vi "4-1.vi"() -> ()   [LabVIEW 2022 SP3, in "AoC22.lvlib"]
uses:
  AoC22.lvlib
  <vilib>/IlluminatedG/lv-stream/Stream.lvlib
panel:
  out "Numeric":i32
  out "Array":i32[][](array[numeric])
  out "sum":i16
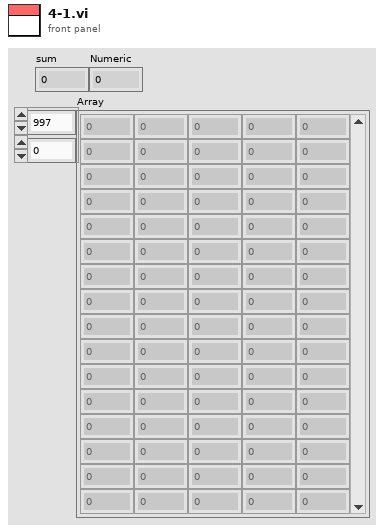
[diagram p1: front panel]
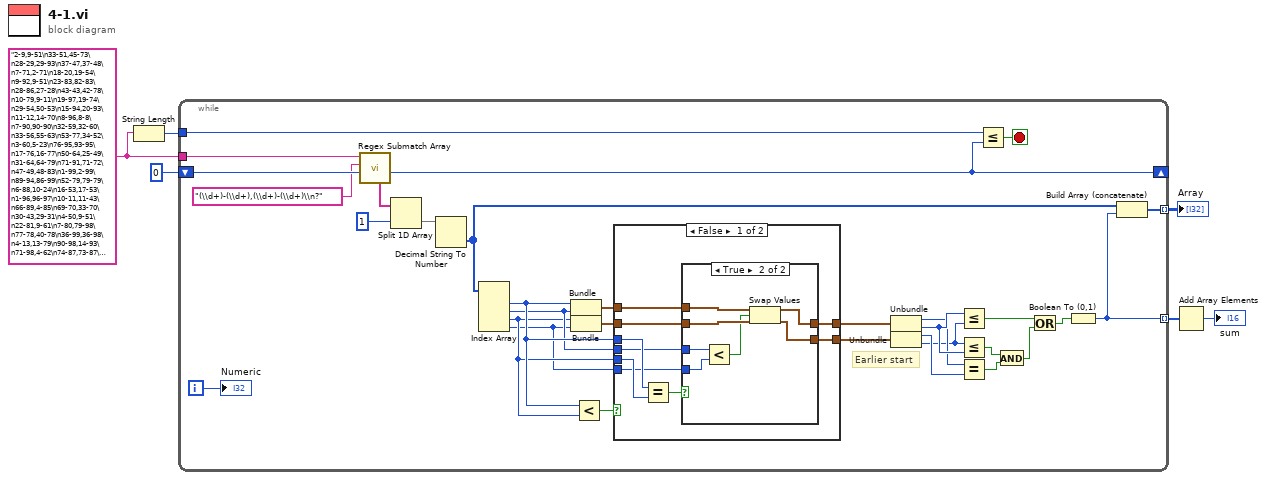
[diagram p0: block diagram]
diagram:
  w5 = "2-9,9-51\n33-51,45-73\n28-29,29-93\n37-47,37-48\n7-71,2-71\n18-20,19-54\n9-92,9-51\n23-83,82-83\n28-86,27-28\n43-43,42-78\n10-79,9-11\n19-97,19-74\n29-54,50-53\n15-94,20-93\n11-12,14-70\n8-96,8-8\n7-90,90-90\n32-59,32-60\n33-56,55-63\n53-77,34-52\n3-60,5-23\n76-95,93-95\n17-76,16-77\n50-64,25-49\n31-64,64-79\n71-91,71-72\n47-49,48-83\n1-99,2-99\n89-94,86-99\n52-79,79-79\n6-88,10-24\n16-53,17-53\n1-96,96-97\n10-11,11-43\n66-89,4-85\n69-70,33-70\n30-43,29-31\n4-50,9-51\n22-81,9-61\n7-80,79-98\n77-78,40-78\n36-99,36-98\n4-13,13-79\n90-98,14-93\n71-98,4-62\n74-87,73-87\n46-86,84-97\n1-57,36-58\n82-96,9-83\n27-96,2-96\n33-33,33-33\n93-94,45-94\n92-92,4-93\n3-70,1-77\n53-94,72-86\n84-85,39-85\n10-74,10-88\n59-95,72-83\n37-75,23-85\n17-19,10-19\n1-83,1-82\n2-93,94-94\n26-84,83-84\n35-57,34-58\n16-74,17-17\n38-88,38-89\n70-96,69-96\n43-76,77-88\n2-99,2-87\n33-56,74-81\n19-50,19-20\n26-94,94-97\n5-78,2-82\n27-77,26-77\n47-98,45-99\n6-89,5-5\n35-56,22-57\n3-96,1-3\n97-97,24-96\n4-35,5-68\n3-5,34-85\n89-90,82-91\n6-46,6-65\n17-34,17-35\n10-82,11-81\n4-53,2-4\n21-88,21-75\n67-99,22-68\n3-89,90-94\n4-97,2-98\n2-69,2-3\n41-62,42-61\n39-88,10-90\n3-43,18-42\n3-83,28-84\n74-87,22-86\n35-98,35-99\n11-92,10-10\n8-15,9-17\n10-17,55-94\n54-74,53-60\n3-96,3-4\n5-18,5-70\n6-88,3-3\n98-98,5-99\n60-87,59-84\n28-76,27-77\n17-26,26-70\n4-6,3-5\n83-99,83-97\n10-65,65-69\n6-73,2-74\n44-96,44-95\n89-89,10-88\n2-91,95-96\n13-60,12-59\n6-29,5-27\n57-57,12-58\n48-85,48-85\n97-98,20-85\n62-97,99-99\n3-6,8-99\n20-34,12-14\n18-84,17-85\n5-88,4-46\n63-67,32-64\n52-80,52-80\n35-97,3-9\n35-78,35-79\n42-65,66-66\n30-30,30-93\n35-44,36-41\n26-95,4-92\n5-5,5-30\n15-88,16-87\n14-54,55-55\n8-41,41-57\n11-93,20-84\n7-61,6-7\n16-37,37-89\n36-89,35-90\n9-39,9-40\n79-92,72-80\n39-97,97-98\n75-81,21-76\n3-70,71-71\n2-94,2-94\n4-5,5-80\n2-84,2-84\n44-57,45-56\n36-76,3-77\n48-54,53-98\n14-71,3-71\n18-98,2-98\n29-85,14-30\n5-88,4-6\n54-84,22-53\n11-75,61-79\n73-74,39-73\n61-98,61-62\n1-4,5-59\n66-94,88-94\n32-38,38-64\n4-59,1-5\n25-57,24-36\n45-69,46-68\n53-77,53-63\n1-94,4-93\n17-89,88-90\n9-90,21-39\n9-90,8-15\n65-82,66-81\n7-83,7-83\n24-98,24-77\n1-1,3-99\n16-18,17-47\n31-87,32-88\n96-98,34-95\n32-67,31-67\n16-58,57-57\n37-83,24-40\n4-66,3-66\n36-74,44-73\n22-81,22-23\n2-7,7-61\n20-21,21-76\n74-74,7-73\n12-46,4-11\n95-99,16-96\n38-80,39-39\n1-19,7-65\n39-53,39-84\n24-82,23-28\n43-44,43-92\n48-60,49-94\n66-85,31-65\n30-31,30-64\n56-95,36-55\n68-93,58-68\n47-59,46-46\n12-33,32-97\n57-75,62-84\n7-8,12-93\n42-75,76-76\n33-81,34-80\n4-5,4-97\n56-78,23-95\n53-53,54-67\n6-46,10-77\n55-87,87-88\n63-83,63-63\n1-1,1-43\n80-92,49-92\n95-99,11-95\n31-34,36-46\n25-83,84-96\n2-98,3-98\n1-3,2-69\n83-97,52-97\n35-93,37-78\n15-44,45-45\n1-99,2-99\n65-89,8-95\n23-59,28-60\n94-94,18-93\n3-44,12-90\n14-51,5-51\n13-38,12-14\n50-88,49-89\n46-69,47-47\n38-44,44-53\n11-73,87-88\n3-58,2-3\n42-89,90-98\n5-41,6-36\n48-90,47-49\n14-50,14-50\n16-24,3-16\n40-41,40-48\n37-37,1-38\n6-38,26-38\n8-96,17-95\n13-98,99-99\n2-57,3-56\n3-30,1-37\n4-68,4-67\n17-20,21-90\n13-17,16-23\n24-25,25-92\n2-2,1-96\n19-91,90-93\n6-79,7-50\n27-28,22-28\n12-98,9-98\n1-4,3-71\n10-20,19-51\n15-15,15-66\n95-95,30-96\n1-93,3-90\n41-43,42-86\n77-93,76-77\n87-99,96-99\n1-99,98-98\n13-70,2-64\n66-84,51-67\n24-89,43-92\n3-43,2-4\n46-48,47-82\n6-96,1-5\n13-76,13-76\n1-83,84-96\n42-60,3-21\n10-49,5-16\n42-95,96-97\n35-35,32-34\n5-7,6-27\n6-16,30-46\n98-99,14-97\n23-75,22-24\n16-18,17-90\n72-73,57-71\n13-78,10-98\n57-62,58-66\n22-57,58-58\n2-75,5-72\n7-24,11-66\n37-91,68-90\n57-94,6-93\n57-67,57-68\n6-18,17-85\n10-10,11-73\n19-35,34-34\n13-30,29-71\n78-78,68-79\n40-54,40-40\n14-60,13-60\n6-31,31-94\n25-76,55-75\n76-81,47-81\n34-58,43-57\n16-60,15-17\n95-97,9-96\n6-7,7-87\n99-99,3-98\n13-36,28-69\n13-26,12-26\n17-57,56-58\n20-95,27-44\n81-88,81-88\n29-45,28-45\n71-77,71-78\n4-17,28-82\n75-77,12-76\n40-44,39-41\n60-90,89-89\n28-43,28-48\n8-89,74-90\n1-4,6-77\n7-74,75-75\n84-94,6-93\n94-95,21-95\n10-63,64-87\n23-97,25-83\n11-68,11-74\n41-45,40-44\n30-88,83-87\n26-74,67-68\n2-6,7-60\n41-41,31-37\n91-91,20-90\n8-8,7-77\n66-77,74-77\n89-97,92-99\n63-70,64-70\n95-98,3-96\n14-79,78-78\n58-81,80-92\n59-94,58-58\n12-23,13-83\n9-85,9-9\n13-97,9-92\n56-73,16-57\n2-96,99-99\n31-73,30-41\n17-91,18-90\n74-94,64-75\n8-97,1-4\n6-95,5-6\n94-97,38-95\n9-80,53-69\n8-8,8-70\n11-94,11-93\n38-86,87-93\n7-85,6-7\n3-90,1-98\n18-88,14-73\n7-95,8-94\n27-77,7-26\n55-98,55-56\n49-90,85-91\n14-64,14-37\n91-95,8-92\n48-94,10-48\n95-96,68-95\n84-98,82-84\n69-69,13-68\n23-93,11-24\n8-25,25-30\n15-79,14-16\n2-98,1-97\n60-70,59-70\n11-69,68-74\n56-83,32-82\n18-97,18-97\n30-72,57-71\n10-55,14-69\n9-9,9-96\n20-92,6-19\n17-47,19-73\n51-86,85-85\n94-94,3-95\n1-99,99-99\n19-22,18-22\n51-76,50-52\n99-99,19-98\n95-95,24-46\n35-81,36-66\n25-86,29-87\n6-50,4-94\n12-35,56-70\n15-69,70-70\n6-95,96-97\n84-97,75-96\n10-10,10-10\n2-22,13-23\n43-90,91-91\n2-95,1-3\n25-65,25-25\n3-57,3-21\n50-64,38-50\n9-94,93-96\n6-49,7-48\n69-82,73-83\n74-95,71-95\n8-95,9-94\n36-78,37-77\n29-31,30-86\n7-78,26-77\n66-66,38-67\n43-86,44-92\n29-31,30-84\n15-59,58-84\n1-1,3-98\n14-33,20-34\n80-80,45-79\n35-95,23-73\n14-16,15-56\n3-56,1-57\n5-98,98-98\n80-93,13-90\n49-96,95-98\n2-85,1-84\n36-43,35-79\n4-99,2-99\n29-94,29-94\n1-95,96-96\n42-47,43-91\n35-98,31-39\n48-71,14-36\n10-70,71-99\n3-3,3-52\n89-89,58-88\n2-91,1-92\n60-82,40-61\n49-50,49-91\n97-97,1-94\n9-9,9-45\n1-1,3-40\n1-99,8-98\n61-63,60-63\n11-38,38-59\n8-54,3-5\n72-80,72-79\n30-97,30-96\n1-99,2-99\n14-62,49-61\n15-28,14-54\n20-27,27-87\n5-55,5-97\n1-94,69-94\n95-98,16-96\n62-62,61-76\n2-10,4-53\n8-73,7-73\n4-87,94-97\n10-82,10-84\n11-77,77-78\n6-98,6-6\n44-63,44-52\n58-90,57-58\n15-79,16-79\n3-8,4-72\n7-17,8-49\n19-87,18-20\n94-94,14-95\n47-65,66-66\n82-97,82-82\n2-11,6-12\n34-36,18-73\n1-30,27-31\n5-97,4-91\n33-83,9-33\n21-73,72-74\n9-75,8-89\n3-6,5-93\n3-77,1-4\n4-31,8-92\n42-50,41-51\n72-89,60-85\n86-89,14-85\n13-72,12-72\n67-79,37-79\n97-99,9-97\n9-50,8-88\n44-65,44-44\n47-78,79-91\n24-64,12-32\n8-83,9-82\n18-85,5-86\n4-69,5-70\n5-91,7-98\n17-19,4-19\n80-80,1-81\n1-95,4-94\n1-69,4-34\n58-59,58-62\n83-95,30-84\n2-30,3-91\n11-30,29-61\n5-94,8-93\n8-12,12-96\n78-95,36-79\n15-87,83-88\n84-84,84-84\n8-10,9-81\n79-98,26-98\n2-2,2-94\n62-78,46-62\n2-79,1-3\n73-75,3-73\n52-54,35-53\n46-81,4-82\n9-96,9-9\n68-98,97-99\n29-74,6-30\n31-31,32-67\n2-97,1-3\n43-47,17-44\n31-75,69-86\n60-72,23-71\n10-67,10-68\n61-63,4-62\n26-65,50-65\n9-29,35-88\n14-78,15-78\n4-76,77-90\n32-33,64-78\n52-92,53-97\n29-47,24-45\n52-70,53-69\n96-96,15-97\n52-89,46-89\n3-5,6-84\n12-75,12-81\n46-57,28-46\n53-76,14-57\n18-52,52-89\n33-53,71-92\n12-28,29-67\n3-7,4-52\n50-55,55-66\n63-63,63-92\n12-86,12-86\n44-57,43-44\n2-61,3-61\n56-85,1-57\n4-6,6-98\n1-75,56-75\n58-60,59-59\n4-22,15-23\n4-17,2-4\n1-33,2-32\n10-89,20-90\n8-72,2-73\n10-69,10-45\n65-80,50-80\n22-94,22-75\n24-98,24-99\n23-99,26-98\n6-71,1-83\n4-5,4-97\n5-25,14-43\n23-74,22-87\n89-96,97-99\n41-46,26-45\n20-86,20-95\n9-97,9-96\n74-77,30-82\n56-68,58-69\n7-10,7-94\n2-87,87-93\n49-92,72-91\n13-14,13-72\n37-38,37-39\n56-74,7-73\n17-95,51-99\n10-95,10-10\n1-97,96-98\n23-53,27-69\n29-65,29-58\n32-89,31-32\n25-43,25-26\n60-61,61-91\n87-89,33-88\n35-35,35-37\n11-47,39-62\n50-52,28-51\n65-65,20-64\n34-91,40-59\n10-67,99-99\n5-82,4-6\n11-40,11-11\n17-57,1-18\n21-22,21-93\n6-79,6-7\n1-75,75-92\n3-82,4-70\n29-58,29-82\n33-33,33-62\n25-33,24-25\n8-80,9-9\n45-69,44-64\n13-17,17-37\n2-97,2-98\n13-88,12-14\n3-61,16-69\n4-95,1-2\n43-45,44-81\n24-71,70-70\n55-92,91-97\n93-98,20-92\n51-52,36-52\n1-97,20-98\n1-86,1-86\n41-85,86-97\n26-28,26-29\n11-38,10-39\n32-70,31-31\n29-31,30-86\n68-94,84-94\n14-19,19-71\n39-94,94-97\n20-41,40-51\n3-88,89-98\n65-86,79-85\n38-99,38-39\n64-75,64-65\n90-92,6-91\n4-30,6-29\n3-47,2-48\n72-85,71-81\n64-70,65-65\n26-95,4-26\n7-13,13-91\n13-81,26-80\n7-67,1-7\n41-58,58-81\n2-96,2-83\n80-89,6-88\n3-41,40-88\n36-46,47-85\n43-81,42-42\n50-50,50-93\n79-91,8-74\n17-24,19-49\n63-80,71-80\n37-91,90-95\n48-90,47-51\n22-79,22-23\n35-57,67-89\n31-54,8-91\n44-68,52-90\n7-75,74-90\n50-64,49-49\n1-1,3-98\n9-98,10-98\n59-91,14-92\n28-93,21-27\n11-81,4-92\n14-21,38-57\n56-90,57-71\n16-67,16-67\n23-56,8-55\n9-47,25-96\n69-96,64-84\n73-78,72-74\n5-48,42-59\n18-53,4-19\n9-23,2-23\n90-92,42-91\n11-39,12-81\n1-93,1-92\n94-98,26-95\n2-10,10-69\n94-94,43-93\n51-97,50-52\n14-35,3-15\n26-26,26-26\n1-96,1-2\n22-84,21-23\n5-82,18-99\n27-37,27-44\n9-10,9-92\n43-88,1-87\n74-74,53-75\n26-96,20-93\n26-70,27-29\n56-60,55-55\n5-89,2-89\n36-88,36-88\n80-80,26-80\n3-3,4-91\n13-18,17-96\n14-43,9-44\n41-69,70-70\n7-93,7-88\n50-51,50-93\n62-62,62-62\n2-93,87-99\n69-98,99-99\n23-24,23-50\n34-65,34-80\n12-25,11-26\n87-88,87-87\n87-91,28-88\n31-33,32-93\n25-38,26-73\n88-97,58-89\n6-96,5-7\n8-56,7-30\n40-91,92-92\n22-24,37-94\n77-83,84-84\n67-67,34-68\n17-19,18-93\n74-97,4-96\n9-87,88-88\n47-48,47-99\n69-69,69-92\n29-68,29-38\n27-29,28-92\n66-78,12-63\n79-82,78-87\n62-67,7-68\n16-92,17-91\n34-79,80-94\n8-36,20-97\n62-77,61-61\n74-81,81-90\n88-90,2-89\n68-91,67-92\n21-24,25-87\n9-63,8-64\n61-79,25-60\n24-51,52-52\n3-89,97-97\n30-94,16-98\n12-74,9-86\n11-91,12-90\n2-4,5-14\n7-91,52-97\n10-58,7-11\n27-66,26-28\n54-81,9-82\n14-59,13-59\n62-62,53-61\n7-15,8-22\n2-8,1-73\n20-65,20-65\n52-52,53-53\n76-85,76-86\n5-11,5-5\n10-72,72-79\n23-92,24-92\n66-97,48-65\n2-69,97-98\n4-51,51-89\n11-95,12-95\n79-98,68-79\n14-22,21-87\n11-53,10-52\n1-74,73-75\n88-92,87-87\n4-91,3-5\n35-91,14-85\n58-91,58-90\n30-30,29-30\n14-49,6-50\n29-78,29-79\n33-62,25-32\n15-92,15-97\n63-70,13-70\n16-81,17-81\n77-77,25-76\n10-72,10-71\n4-79,2-5\n15-21,15-46\n41-58,26-57\n10-62,63-87\n12-24,24-71\n5-58,59-59\n11-15,10-10\n44-61,43-47\n74-74,7-73\n3-85,86-93\n29-56,30-55\n33-40,25-39\n37-69,69-80\n25-89,12-88\n6-99,5-6\n8-10,9-73\n31-47,46-80\n57-57,3-56\n65-65,13-66\n3-85,1-97\n78-92,40-77\n45-64,38-63\n12-13,13-99\n84-92,83-91\n73-91,74-74\n23-55,2-24\n16-52,15-53\n12-29,29-78\n96-98,12-96\n82-89,88-88\n59-78,50-64\n9-9,9-63\n15-47,14-16\n42-72,20-65\n41-92,13-93\n78-85,70-79\n25-53,20-24\n62-96,61-63\n50-57,49-58\n14-93,14-95\n3-10,2-10\n84-84,77-83\n1-99,1-2\n50-90,36-91\n95-95,6-94\n29-38,29-49\n31-89,31-31\n5-81,4-76\n47-74,58-73\n69-90,68-68\n15-80,12-16\n53-85,84-86\n18-24,19-25\n14-16,15-88\n13-90,2-97\n90-91,90-90\n52-54,17-53\n50-59,43-52\n21-59,54-60\n64-84,64-82\n64-64,38-63\n43-75,69-73\n30-56,55-57\n46-63,39-46\n3-96,96-96\n1-97,15-93\n20-62,20-20\n65-90,64-79\n94-94,12-93\n45-53,13-46\n21-89,22-88\n18-31,32-38\n48-68,47-70\n29-92,30-91\n20-58,20-20\n66-66,66-95\n39-67,24-40\n8-95,4-96\n27-75,65-85\n1-94,93-93\n77-93,92-97\n53-54,52-55\n37-62,36-37\n7-11,6-61\n34-62,35-61\n54-56,55-57\n60-60,61-73\n48-66,64-76\n59-73,38-60\n3-8,3-97\n93-93,79-92\n4-40,39-40\n80-87,8-81\n7-22,21-88\n2-97,13-99\n33-99,32-81\n45-82,23-82\n34-91,34-35\n76-81,50-80\n9-76,76-97\n33-90,33-33\n32-59,31-59\n1-91,3-90\n60-97,96-99\n89-89,3-90\n10-36,6-11\n41-92,48-90\n26-87,70-88\n73-74,74-86\n16-77,15-16\n4-95,1-4\n77-93,76-98\n74-75,45-75\n8-60,8-56\n4-98,2-31\n16-87,86-98\n25-73,72-74\n27-88,26-89\n13-35,11-60\n75-75,71-76\n56-96,95-97\n14-86,15-39\n15-35,16-35\n78-78,29-77\n32-92,54-92\n3-32,31-67\n66-85,66-66\n10-61,9-10\n34-81,35-89\n8-83,98-99\n3-99,3-4\n18-38,19-37\n19-19,19-33\n15-69,14-70\n11-72,11-87\n42-65,40-76\n8-55,16-29\n3-11,10-82\n12-76,14-89\n40-51,12-65\n11-93,11-94\n1-76,1-77\n83-89,48-87\n8-67,7-51\n77-82,77-81\n18-80,19-81\n32-42,43-65\n20-40,16-20\n22-82,22-83\n92-93,45-92\n44-46,45-98\n13-95,13-14\n45-72,46-72\n1-94,37-99\n51-84,12-83\n33-99,34-98\n5-6,5-57\n9-80,8-81\n54-66,44-52\n31-36,14-98\n56-60,57-60\n2-46,47-47\n6-13,16-19\n88-88,14-89\n95-96,20-95\n32-97,70-97\n33-41,33-47\n1-99,2-98\n1-60,55-60\n67-68,52-68\n13-88,3-14\n27-36,41-50\n44-75,75-76\n18-57,56-96\n21-71,22-72\n6-50,5-7\n3-79,2-4\n31-84,56-90\n6-97,9-97\n24-96,23-23\n21-22,21-21\n18-84,3-76\n43-57,44-63\n5-5,3-6\n68-98,57-94\n14-69,15-68\n48-62,48-86\n52-95,75-92\n33-58,32-76\n11-28,7-12\n42-42,42-97\n42-44,43-90\n27-97,98-99\n5-63,5-5\n68-74,59-74\n1-3,4-60\n15-53,6-14\n27-45,26-46\n36-93,15-94\n64-85,40-66\n26-53,43-52\n3-93,2-26\n7-99,11-97\n12-96,13-98\n16-84,7-17\n15-16,15-93\n21-93,45-93\n45-46,46-47\n58-65,57-65\n5-98,38-97\n19-33,25-38\n21-81,16-69\n48-88,75-79\n88-99,64-97\n5-71,2-72\n16-80,15-80\n1-3,2-99\n38-92,37-38\n58-79,45-73\n27-91,27-27\n24-67,22-22\n14-48,13-20\n4-4,3-34\n15-15,14-51\n7-20,6-21"
  n1 = String Length(string=w5) -> (length=w4:i32)
  n2 = while {
    tunnel: w5 -> [w37]
    shift-right: [w35] -> _
    shift-left: 0 -> [w36]
    tunnel: w4 -> [w34]
    tunnel: [w18] -> w2 mode=indexing
    tunnel: [w17] -> w1 mode=indexing
    i -> [w16]
    stop <- w33 stop-if-true
    # "Earlier start"
    n3 = call <vilib>:"Regex Submatch Array.vi"("offset (0)"=w36, "regular expression"="(\\d+)-(\\d+),(\\d+)-(\\d+)\\n?", "string"=w37) -> ("offset past match"=w35:i32, "matches"=w31:string[])  [unwired: 6 in, 1 out]
    n4 = Split 1D Array(array=w31, index=1) -> (second subarray=w29:string[])  [unwired: 1 out]
    n5 = Decimal String To Number(string=w29) -> (number=w20:i32[])  [unwired: 2 in, 1 out]
    n6 = Index Array(array=w20) -> (element #1=w10:i32, element #2=w9:i32, element #3=w8:i32, element #4=w7:i32)  [unwired: 4 in]
    n7 = Bundle("String"=w10, "String"=w9) -> (w13:cluster{"String":i32, "String":i32})  [unwired: 1 in]
    n8 = Bundle("String"=w8, "String"=w7) -> (w14:cluster{"String":i32, "String":i32})  [unwired: 1 in]
    n9 = Less?(x=w10, y=w8) -> (x < y?=w15:bool)
    n10 = case shown="False" w15 {
      tunnel: w14 -> [w43 w56]
      tunnel: w13 -> [w41 w57]
      tunnel: [w42 w57] -> w12
      tunnel: [w40 w56] -> w11
      tunnel: w10 -> [w46 _]
      tunnel: w9 -> [w39 _]
      tunnel: w8 -> [w45 _]
      tunnel: w7 -> [w38 _]
      frame False {
        n11 = Equal?(x=w46, y=w45) -> (x = y?=w44:bool)
        n12 = case shown="True" w44 {
          tunnel: w43 -> [w48 w52]
          tunnel: [w48 w50] -> w42
          tunnel: w41 -> [w47 w53]
          tunnel: [w47 w49] -> w40
          tunnel: w39 -> [_ w55]
          tunnel: w38 -> [_ w54]
          frame False {
          }
          frame True {
            n13 = Less?(x=w55, y=w54) -> (x < y?=w51:bool)
            n14 = Swap Values(12:w53, 13:w51, 14:w52) -> (1:w49:cluster{"String":i32, "String":i32}, 3:w50:cluster{"String":i32, "String":i32})
          }
        }
      }
      frame True {
      }
    }
    n15 = Unbundle(w11) -> ("String"=w22:i32, "String"=w26:i32)
    n16 = Unbundle(w12) -> ("String"=w27:i32, "String"=w21:i32)
    n17 = Less Or Equal?(x=w26, y=w21) -> (x <= y?=w28:bool)
    n18 = Less Or Equal?(x=w21, y=w26) -> (x <= y?=w25:bool)
    n19 = Equal?(x=w22, y=w27) -> (x = y?=w24:bool)
    n20 = Less Or Equal?(x=w34, y=w35) -> (x <= y?=w33:bool)
    n21 = And(x=w25, y=w24) -> (x .and. y?=w23:bool)
    n22 = Or(x=w28, y=w23) -> (x .or. y?=w19:bool)
    n23 = Boolean To (0,1)(Boolean=w19) -> (0, 1=w17:i16)
    n24 = Build Array (concatenate)(w20, w17) -> (w18:i32[])
    "Numeric" <- w16
  }
  "Array" <- w2
  n25 = Add Array Elements(numeric array=w1) -> (sum=→"sum":i16)
